vi "RFH-View-sort_by_name.vi"() -> ()   [LabVIEW 2020, in "RFH-Reflection_File_Handler.lvlib"]
uses:
  RFH-Reflection_File_Handler.lvlib
  RFH-common_data_format.ctl
  <vilib>/Comparison/Less/Less Functor/Less Functor.lvclass
  c8c21ec7-ed02-4f39-bd47-49b2af03b8e9.vi
panel:
  out "sorted array":string[](array[string])
  out "Array":string[](array[string])
  out "Reflection Imag 2":T1(graph)
  in  "stop":bool
  out "Reflection Imag":T1(graph)
  in  "Folder Path":path=path "C:/projects/Universitet/Master/data/Real Test - First libreVNA test with calibration file/Converted Data"
  out "Reflection Real":T1(graph)
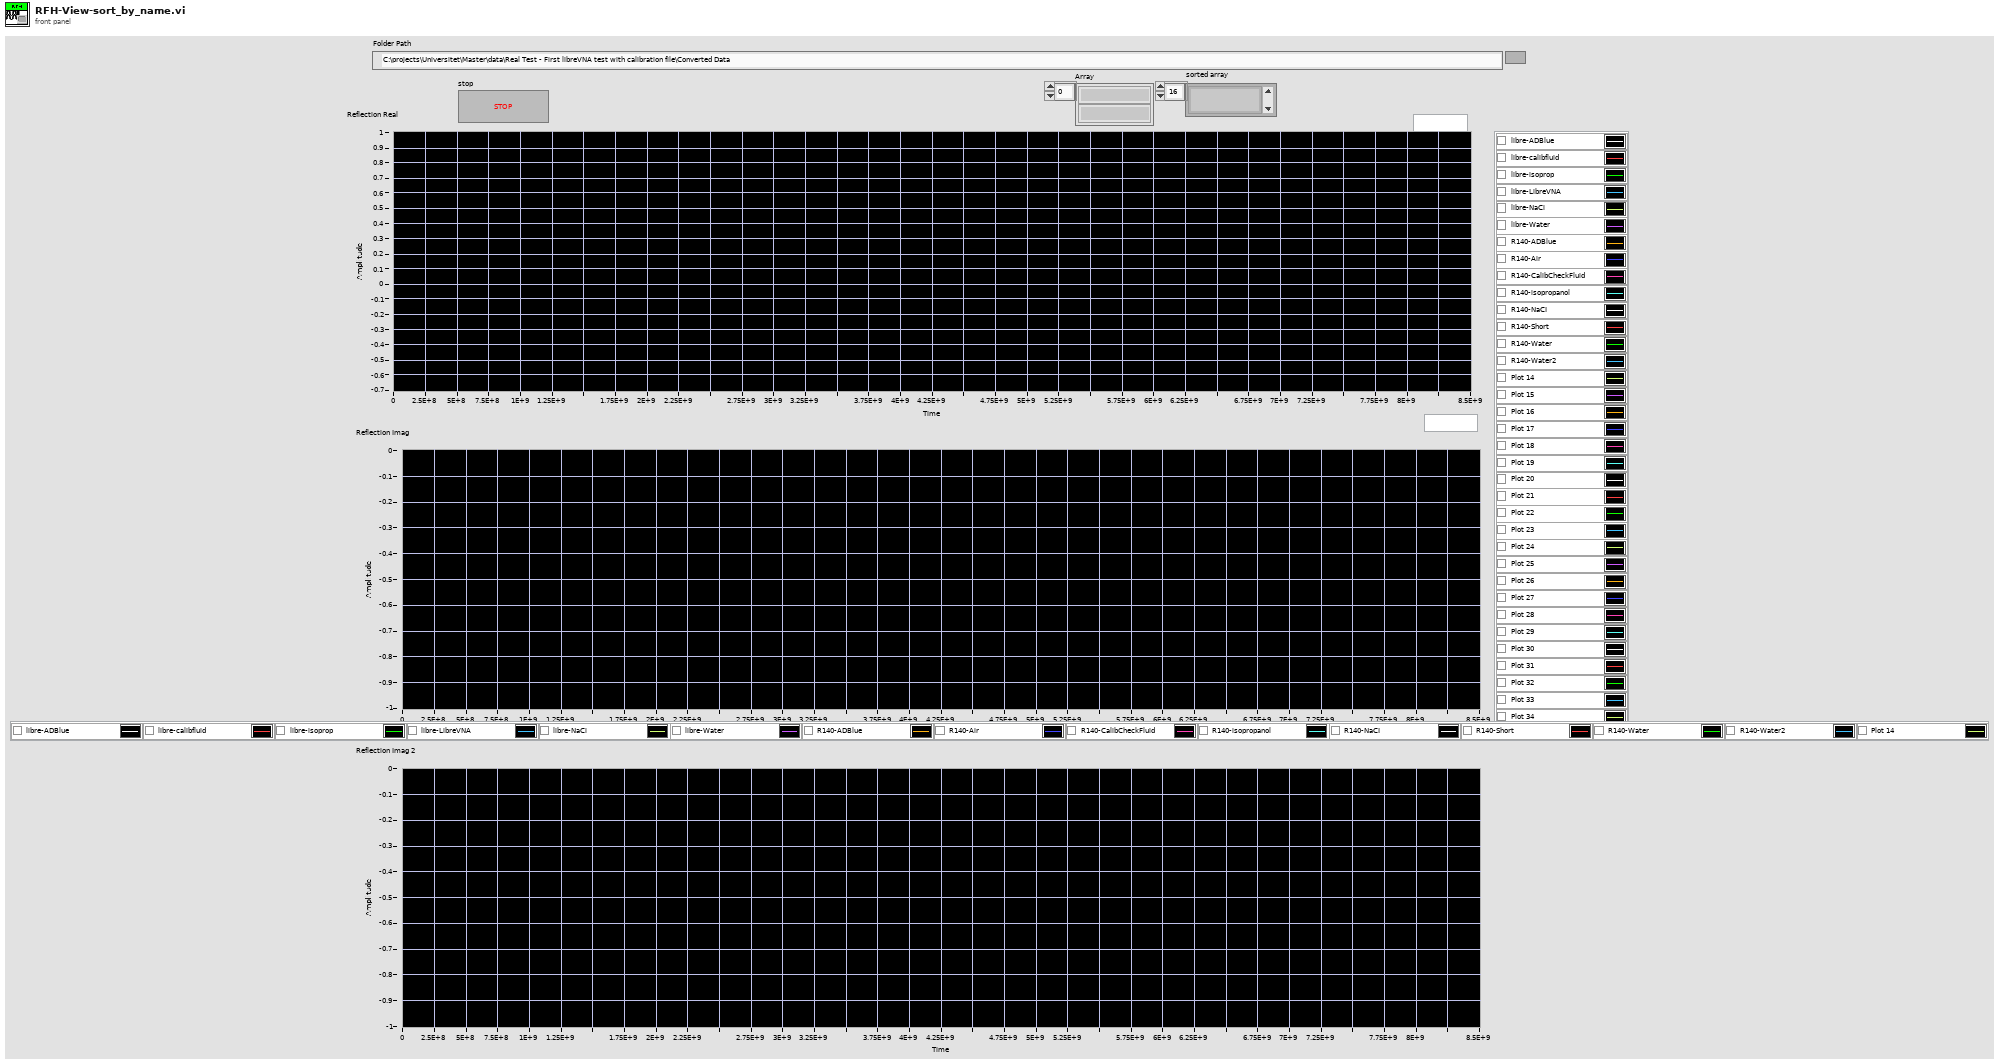
[diagram p1: front panel]
types:
  T1 = cluster{"Frequency":dbl[], "Reflection'":dbl[]}[]
  T2 = typedef "RFH-Reflection_File_Handler.lvlib/RFH-common_data_format.ctl" = cluster{"Frequency":dbl[], "Reflection'":dbl[], "Reflection''":dbl[], "Permativity'":dbl[], "Permativity''":dbl[]}
  T3 = cluster{"filename without extension":string, "Common Format":T2}
  T4 = map{string, cluster{"filename without extension":string, "Common Format":T2}}
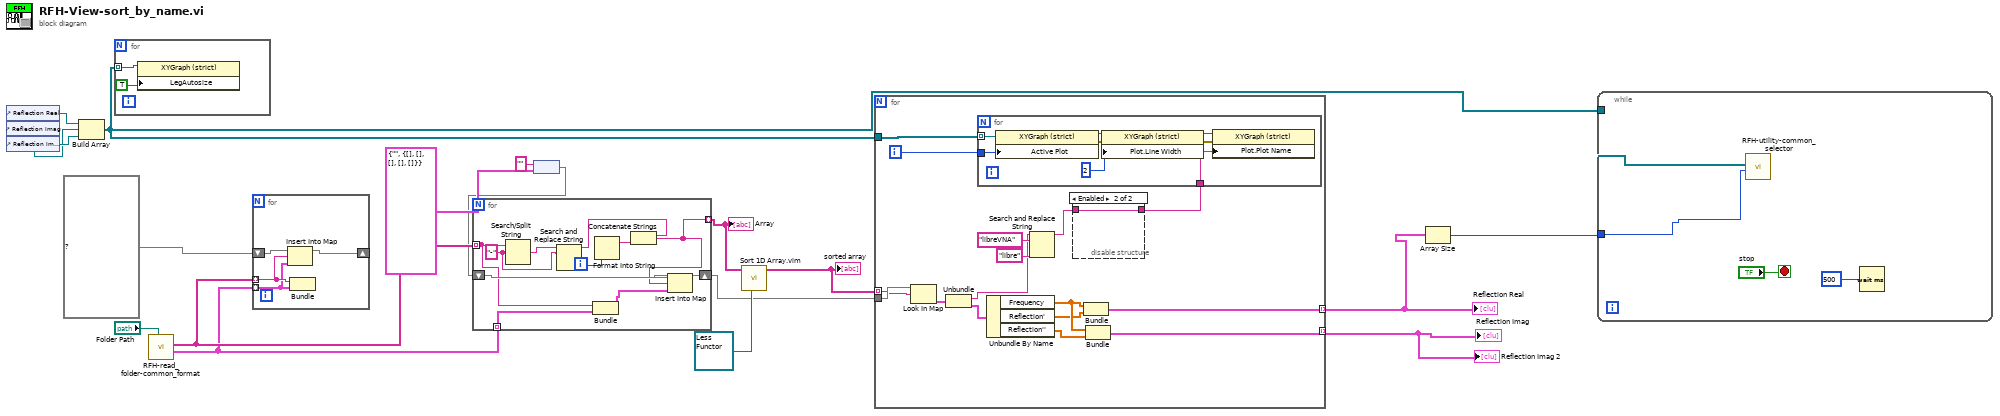
[diagram p0: block diagram]
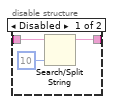
[diagram p2: hidden frame]
diagram:
  n1 = control-ref of="Reflection Real"() -> (w14:refnum<vi>)
  n2 = control-ref of="Reflection Imag"() -> (w13:refnum<vi>)
  n3 = control-ref of="Reflection Imag 2"() -> (w15:refnum<vi>)
  n4 = Build Array(w14, w13, w15) -> (w17:refnum<vi>[])
  n5 = for {
    tunnel: w17 -> [w19] mode=indexing
    n6 = property on="Property Node" class="XYGraph (strict)"(reference=w19, "LegAutosize"=TRUE ("Legend:Autosize")) -> ()  [unwired: 1 in, 2 out]
  }
  n7 = call "RFH-read_folder-common_format.vi"("Folder Path"="Folder Path") -> ("Data"=w8:T2[], "Names"=w9:string[])  [unwired: 9 in]
  n8 = for {
    tunnel: w9 -> [w23] mode=indexing
    tunnel: w8 -> [w22] mode=indexing
    shift-right: [w21] -> _
    shift-left: map{string, T2} {} ("map") -> [w24]
    n9 = Insert Into Map(map in=w24, key=w23, value=w22) -> (map out=w21:map{string, T2})  [unwired: 2 out]
    n10 = Bundle("filename without extension"=w23, "Common Format"=w22) -> ()  [unwired: 1 in, 1 out]
  }
  n11 = node("" ("key"), T3 {"filename without extension"="", "Common Format"={"Frequency"=[], "Reflection'"=[], "Reflection''"=[], "Permativity'"=[], "Permativity''"=[]}} ("output cluster")) -> (w5:T4)
  n12 = for {
    tunnel: w9 -> [w26] mode=indexing
    tunnel: [w25] -> w4 mode=indexing
    tunnel: w8 -> [w33] mode=indexing
    shift-right: [w30] -> w1
    shift-left: w5 -> [w32]
    i -> [w29]
    w34 = "-" ("search string/char (-)")
    n13 = Search/Split String(string=w26, search string/char (-)=w34) -> (match + rest of string=w35:string)  [unwired: 1 in, 2 out]
    n14 = Search and Replace String(input string=w35, search string=w34) -> (result string=w28:string)  [unwired: 6 in, 3 out]
    n15 = Bundle("filename without extension"=w26, "Common Format"=w33) -> (w31:T3)  [unwired: 1 in]
    n16 = Format Into String(w29) -> (resulting string=w27:string)  [unwired: 3 in, 1 out]
    n17 = Concatenate Strings(w28, w27) -> (w25:string)
    n18 = Insert Into Map(map in=w32, key=w25, value=w31) -> (map out=w30:T4)  [unwired: 2 out]
  }
  "Array" <- w4
  n19 = call "Sort 1D Array.vim"("less function (built-in <)"=refnum<class "Less Functor.lvclass"> refnum, "unsorted array"=w4) -> ("sorted array"=w2:string[])  [unwired: 9 in]
  "sorted array" <- w2
  n20 = for {
    tunnel: [w48] -> w12 mode=indexing
    tunnel: [w47] -> w16 mode=indexing
    tunnel: w17 -> [w41]
    tunnel: w2 -> [w39] mode=indexing
    tunnel: w1 -> [w40]
    i -> [w46]
    n21 = Look In Map(map=w40, key=w39) -> (value=w38:T3)  [unwired: 1 in, 1 out]
    n22 = Unbundle(w38) -> ("filename without extension"=w37:string, "Common Format"=w36:T2)
    n23 = Unbundle By Name(w36) -> ("Frequency"=w51:dbl[], "Reflection'"=w50:dbl[], "Reflection''"=w49:dbl[])
    n24 = Search and Replace String(input string=w37, search string="libreVNA", replace string="libre" ("replace string (\"\")")) -> (result string=w42:string)  [unwired: 5 in, 3 out]
    n25 = disable-structure shown="Enabled" {
      disable-tunnel: [w53 w55] -> w45
      disable-tunnel: w42 -> [w52 w55]
      frame Disabled {
        n26 = Search/Split String(string=w52, offset (0)=10) -> (substring before match=w53:string)  [unwired: 1 in, 2 out]
      }
      frame Enabled {
      }
    }
    n27 = for {
      tunnel: w46 -> [w62]
      tunnel: w45 -> [w59]
      tunnel: w41 -> [w58] mode=indexing
      n28 = property on="Property Node" class="XYGraph (strict)"(reference=w58, "Active Plot"=w62) -> (reference out=w57:refnum<vi>, error out=w63:errorcluster)  [unwired: 1 in]
      n29 = property on="Property Node" class="XYGraph (strict)"(reference=w57, error in=w63, "Plot.Line Width"=u8 2) -> (reference out=w56:refnum<vi>, error out=w61:errorcluster)
      n30 = property on="Property Node" class="XYGraph (strict)"(reference=w56, error in=w61, "Plot.Plot Name"=w59) -> ()  [unwired: 2 out]
    }
    n31 = Bundle("Frequency"=w51, "Reflection'"=w50) -> (w48:cluster{"Frequency":dbl[], "Reflection'":dbl[]})  [unwired: 1 in]
    n32 = Bundle("Frequency"=w51, "Reflection''"=w49) -> (w47:cluster{"Frequency":dbl[], "Reflection''":dbl[]})  [unwired: 1 in]
  }
  "Reflection Real" <- w12
  "Reflection Imag" <- w16
  "Reflection Imag 2" <- w16
  n33 = Array Size(array=w12) -> (size(s)=w11:i32)
  n34 = while {
    tunnel: w17 -> [w67]
    tunnel: w11 -> [w65]
    stop <- "stop" stop-if-true
    n35 = call "RFH-utility-common_selector.vi"("size(s)"=w65, "XY graph refs"=w67) -> ()  [unwired: 10 in]
    n36 = Wait (ms)(milliseconds to wait=u32 500) -> ()  [unwired: 1 out]
  }
